vi "Set Channel Gain.vi"(8 "error in (no error)":errorcluster, 10 "Params":variant, 11 "PI650 VoltageAmp in":refnum<class "PI650 VoltageAmp.lvclass">) -> (0 "error out":errorcluster, 3 "PI650 VoltageAmp out":refnum<class "PI650 VoltageAmp.lvclass">)   [LabVIEW 2020, in "Pickering.lvlib" / "PI650 VoltageAmp.lvclass"]
uses:
  PI650 VoltageAmp.lvclass
  PI650 VoltageAmp.lvclass/PI650 VoltageAmp.ctl
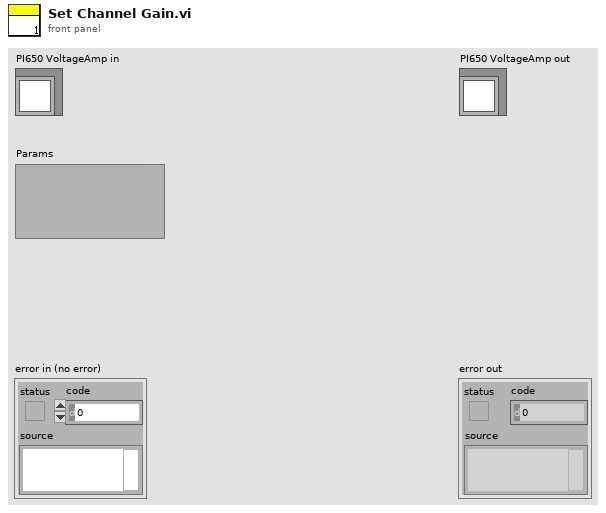
[diagram p1: front panel]
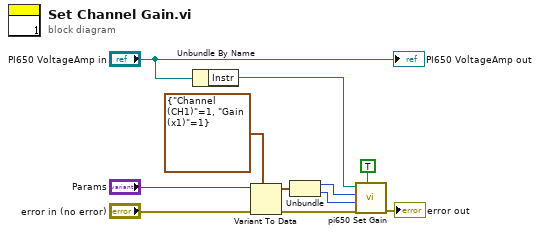
[diagram p0: block diagram]
diagram:
  n1 = Unbundle By Name("PI650 VoltageAmp in") -> ("Instr"=w9:refnum<visa-resource-name>)
  n2 = Variant To Data(error in="error in (no error)", type=cluster{"Channel (CH1)":u32, "Gain (x1)":u32} {"Channel (CH1)"=1, "Gain (x1)"=1}, Variant="Params") -> (data=w4:cluster{"Channel (CH1)":u32, "Gain (x1)":u32}, error out=w8:errorcluster)
  n3 = Unbundle(w4) -> ("Channel (CH1)"=w3:u32, "Gain (x1)"=w2:u32)
  n4 = call <instrlib>:"pi650 Set Gain.vi"("Action (VI_ON)"=TRUE, "error in (no error)"=w8, "Gain (x1)"=w2, "Channel (CH1)"=w3, "instrument handle"=w9) -> ("error out"=→"error out":errorcluster)  [unwired: 5 in, 1 out]
  "PI650 VoltageAmp out" <- "PI650 VoltageAmp in"
